vi "Set Type.vi"(10 "Type":refnum<class "Type.lvclass">, 11 "ColumnPanel in":refnum<class "ColumnPanel.lvclass">) -> (3 "ColumnPanel out":refnum<class "ColumnPanel.lvclass">)   [LabVIEW 2020, in "Conditum-Tools.lvlib" / "ColumnPanel.lvclass"]
uses:
  ColumnPanel.lvclass
  Conditum-Clone/Columns/Type/Type.lvclass
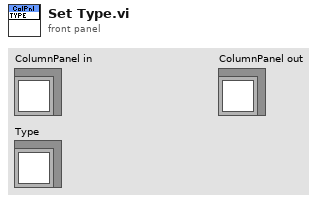
[diagram p1: front panel]
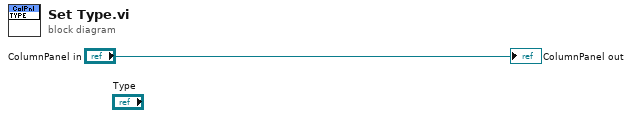
[diagram p0: block diagram]
diagram:
  "ColumnPanel out" <- "ColumnPanel in"
